vi "Write configuration.vi"(8 "error in (no error)":errorcluster, 11 "Tomo in":refnum<class "Tomo.lvclass">) -> (0 "error out":errorcluster, 3 "Tomo out":refnum<class "Tomo.lvclass">)   [LabVIEW 2012, in "Tomo.lvclass"]
doc: "Writes the configuration cluster into the configuration file. Configuration file is XML-based. It's name is <component ID>.xml"
uses:
  Tomo.lvclass
  <vilib>/Distrio/Murmex/Murmex/Murmex.lvclass
  Tomo.lvclass/Tomo.ctl
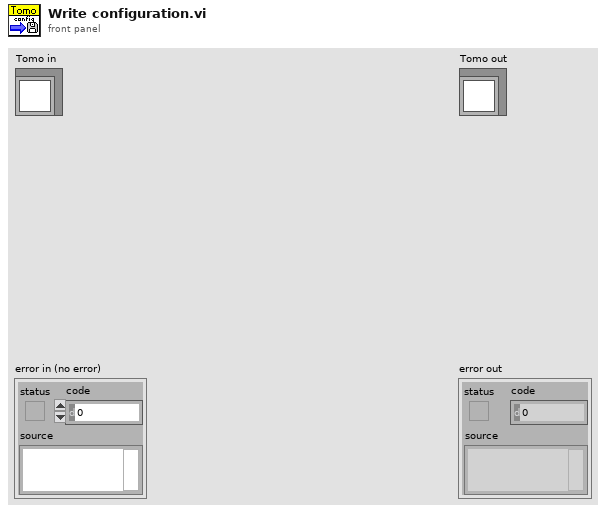
[diagram p1: front panel]
types:
  T1 = typedef "Tomo.lvclass/configuration cluster.ctl" = cluster{"stack component":string, "camera component":string, "stages component":string, "mapping file folder":path, "default stages speed":dbl[unit], "stack overhead time":dbl[unit], "autofocus component":string, "imaging component":string}
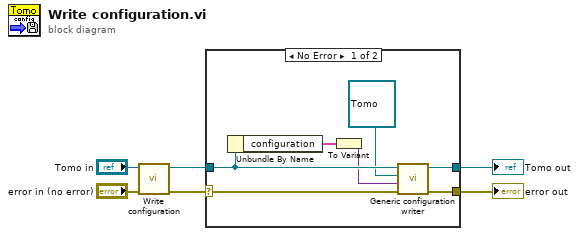
[diagram p0: block diagram]
diagram:
  n1 = call-parent "Write configuration.vi"("error in (no error)"="error in (no error)", "Murmex in"="Tomo in") -> ("error out"=w4:errorcluster, "Murmex out"=w3:refnum<class "Tomo.lvclass">)  [unwired: 8 in]
  n2 = case shown="No Error" w4 {
    selector: w4 -> [w13 w15]
    tunnel: w3 -> [w12 w14]
    tunnel: [w8 w14] -> w2
    tunnel: [w7 w15] -> w1
    frame No Error {
      n3 = Unbundle By Name(w12) -> ("configuration"=w11:T1)
      n4 = To Variant(anything=w11) -> (Variant=w10:variant)
      n5 = call <vilib>:"Generic configuration writer.vi"("error in (no error)"=w13, "configuration"=w10, "inheritance level"=refnum<class "Tomo.lvclass"> refnum ("Tomo.lvclass"), "MurmexBase in"=w12) -> ("error out"=w7:errorcluster, "MurmexBase out"=w8:refnum<class "Tomo.lvclass">)  [unwired: 6 in]
    }
    frame Error {
    }
  }
  "error out" <- w1
  "Tomo out" <- w2
